vi "aft_FXP_LMS_Simulation_Unit.vi"(7 "stepsize":fxp<+/-,64,32>, 8 "d(n)":fxp<+/-,32,32>, 9 "x(n)":fxp<+/-,32,32>, 10 "coefficients in":fxp<+/-,32,32>[](array[numeric]), 11 "state in":fxp<+/-,32,32>[](array[numeric])) -> (0 "e(n)":fxp<+/-,32,32>, 1 "d'(n)":fxp<+/-,32,16>, 2 "coefficients out":fxp<+/-,64,81>[](array[numeric]), 3 "state out":fxp<+/-,32,32>[](array[numeric]), 4 "coefficients overflow":bool)   [LabVIEW 2017]
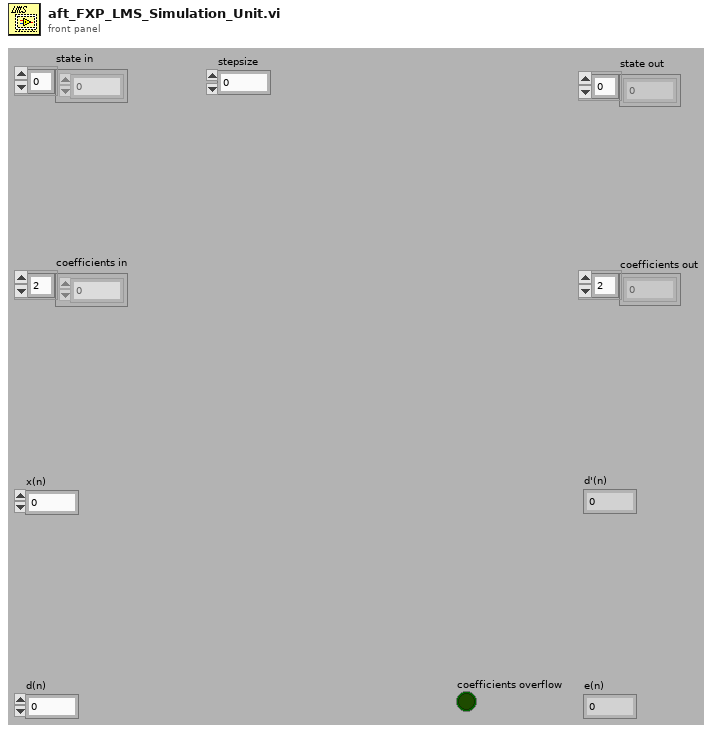
[diagram p1: front panel]
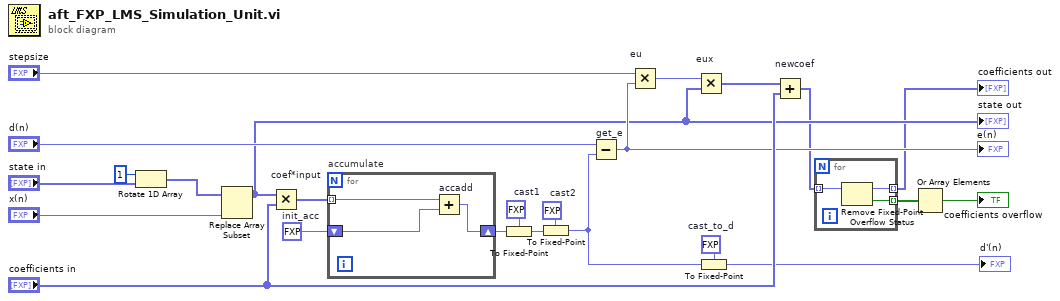
[diagram p0: block diagram]
diagram:
  w1 = fxp<+/-,64,66> 0.0  # cast2
  w4 = fxp<+/-,64,66> 0.0  # cast1
  w9 = fxp<+/-,32,16> 0.0  # cast_to_d
  w15 = fxp<+/-,64,66> 0.0  # init_acc
  n1 = Rotate 1D Array(1:"state in", 2:1 ("n")) -> (0:w17:fxp<+/-,32,32>[])
  n2 = Replace Array Subset(array=w17, new element="x(n)") -> (w18:fxp<+/-,32,32>[])  [unwired: 1 in]
  "state out" <- w18
  n3 = Multiply "coef*input"(x=w18, y="coefficients in") -> (x*y=w10:fxp<+/-,64,64>[])
  n4 = for "accumulate" {
    tunnel: w10 -> [w27] mode=indexing
    shift-right: [w25] -> w5
    shift-left: w15 -> [w26]
    n5 = Add "accadd"(x=w27, y=w26) -> (x+y=w25:fxp<+/-,64,66>)
  }
  n6 = To Fixed-Point(fixed-point type=w4, number=w5) -> (fixed-point=w3:fxp<+/-,64,66>)
  n7 = To Fixed-Point(fixed-point type=w1, number=w3) -> (fixed-point=w2:fxp<+/-,64,66>)
  n8 = Subtract "get_e"(x="d(n)", y=w2) -> (x-y=w20:fxp<+/-,32,32>)
  "e(n)" <- w20
  n9 = Multiply "eu"(x="stepsize", y=w20) -> (x*y=w14:fxp<+/-,64,48>)
  n10 = Multiply "eux"(x=w14, y=w18) -> (x*y=w13:fxp<+/-,64,79>[])
  n11 = To Fixed-Point(fixed-point type=w9, number=w2) -> (fixed-point=→"d'(n)":fxp<+/-,32,16>)
  n12 = Add "newcoef"(x=w13, y="coefficients in") -> (x+y=w11:fxp<+/-,64,81>[])
  n13 = for {
    tunnel: w11 -> [w30] mode=indexing
    tunnel: [w29] -> w12 mode=indexing
    tunnel: [w28] -> w8 mode=indexing
    n14 = Remove Fixed-Point Overflow Status(3:w30) -> (0:w29:bool, 1:w28:fxp<+/-,64,81>)
  }
  "coefficients out" <- w8
  n15 = Or Array Elements(Boolean array=w12) -> (logical OR=→"coefficients overflow":bool)
